vi "Header_Measureit.vi"(1 "Cluster":T1={"Preamp Bias on?"=FALSE, "Preamp Bias (mv)"=-10, "Preamp Sensitivity"=enum."100nA/V", "Detect Sens?"=TRUE, "Sens Change wait time (ms)"=1000, "Auto-pick min. sensitivity"=enum."100nA/V", "Auto-pick Sens?"=FALSE}, 2 "String in":string) -> (0 "String out":string)   [LabVIEW 2013]
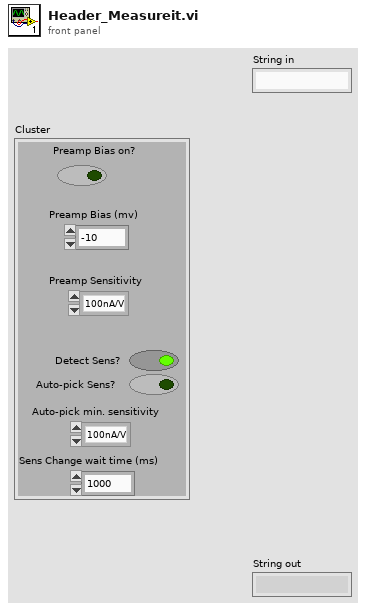
[diagram p1: front panel]
types:
  T1 = cluster{"Preamp Bias on?":bool, "Preamp Bias (mv)":i32, "Preamp Sensitivity":enum16{"1pA/V", "2pA/V", "5pA/V", "10pA/V", "20pA/V", "50pA/V", "100pA/V", "200pA/V", "500pA/V", "1nA/V", "2nA/V", "5nA/V", "10nA/V", "20nA/V", "50nA/V", "100nA/V", "200nA/V", "500nA/V", "1uA/V", "2uA/V", "5uA/V", "10uA/V", "20uA/V", "50uA/V", "100uA/V", "200uA/V", "500uA/V", "1mA/V"}, "Detect Sens?":bool, "Sens Change wait time (ms)":u32, "Auto-pick min. sensitivity":enum16{"1pA/V", "2pA/V", "5pA/V", "10pA/V", "20pA/V", "50pA/V", "100pA/V", "200pA/V", "500pA/V", "1nA/V", "2nA/V", "5nA/V", "10nA/V", "20nA/V", "50nA/V", "100nA/V", "200nA/V", "500nA/V", "1uA/V", "2uA/V", "5uA/V", "10uA/V", "20uA/V", "50uA/V", "100uA/V", "200uA/V", "500uA/V", "1mA/V"}, "Auto-pick Sens?":bool}
  T2 = enum16{"1pA/V", "2pA/V", "5pA/V", "10pA/V", "20pA/V", "50pA/V", "100pA/V", "200pA/V", "500pA/V", "1nA/V", "2nA/V", "5nA/V", "10nA/V", "20nA/V", "50nA/V", "100nA/V", "200nA/V", "500nA/V", "1uA/V", "2uA/V", "5uA/V", "10uA/V", "20uA/V", "50uA/V", "100uA/V", "200uA/V", "500uA/V", "1mA/V"}
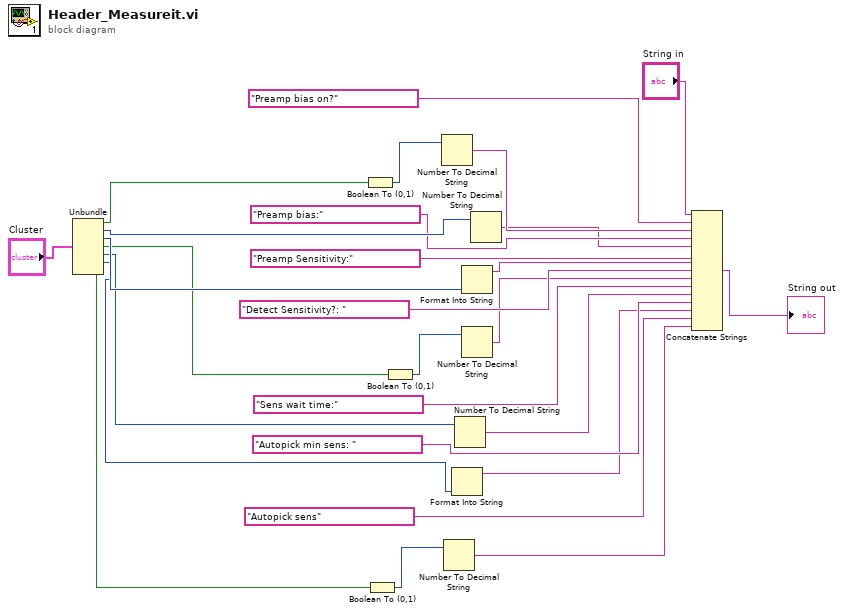
[diagram p0: block diagram]
diagram:
  n1 = Unbundle("Cluster") -> ("Preamp Bias on?"=w26:bool, "Preamp Bias (mv)"=w24:i32, "Preamp Sensitivity"=w23:T2, "Detect Sens?"=w21:bool, "Sens Change wait time (ms)"=w20:u32, "Auto-pick min. sensitivity"=w19:T2, "Auto-pick Sens?"=w17:bool)
  n2 = Boolean To (0,1)(Boolean=w26) -> (0, 1=w25:i16)
  n3 = Boolean To (0,1)(Boolean=w17) -> (0, 1=w18:i16)
  n4 = Boolean To (0,1)(Boolean=w21) -> (0, 1=w22:i16)
  n5 = Number To Decimal String(number=w25) -> (decimal integer string=w13:string)  [unwired: 1 in]
  n6 = Number To Decimal String(number=w18) -> (decimal integer string=w1:string)  [unwired: 1 in]
  n7 = Format Into String(w19) -> (resulting string=w3:string)  [unwired: 3 in, 1 out]
  n8 = Number To Decimal String(number=w20) -> (decimal integer string=w5:string)  [unwired: 1 in]
  n9 = Format Into String(w23) -> (resulting string=w9:string)  [unwired: 3 in, 1 out]
  n10 = Number To Decimal String(number=w22) -> (decimal integer string=w7:string)  [unwired: 1 in]
  n11 = Number To Decimal String(number=w24) -> (decimal integer string=w11:string)  [unwired: 1 in]
  n12 = Concatenate Strings("String in", "Preamp bias on?" ("string"), w13, "Preamp bias:" ("string"), w11, "Preamp Sensitivity:" ("string"), w9, "Detect Sensitivity?: " ("string"), w7, "Sens wait time:" ("string"), w5, "Autopick min sens: " ("string"), w3, "Autopick sens" ("string"), w1) -> (→"String out":string)
